vi "ATE_RVP8_Cal_Attn.vi"() -> ()   [LabVIEW 2009]
doc: "Use this template to build a producer/consumer design pattern with events to produce queue items. Use this design pattern instead of the User Interface Event Handler pattern for user interfaces when you want to execute code asynchronously in response to an event without slowing the user interface responsiveness."
uses:
  Rvp8PowerData.ctl
  <vilib>/Analysis/NI_AALBase.lvlib
  <vilib>/Analysis/NI_AALPro.lvlib
panel:
  in  "Configuration 1":bool
  out "Cal Output File":path
  out "Cal differences":cluster{i32[], dbl[]}[](graph)
  out "RVP8 calibration":cluster{i32[], dbl[]}[](graph)
  in  "DataSource":bool
  out "Cal file name":string
  in  "Cal data directory":string="/home/operator/data/rvp8_cal_attn"
  in  "Set SigGen":bool
  in  "Initialize":bool
  in  "70 dB":bool
  in  "121 dB":bool
  in  "Switches":bool
  in  "Calibrate":bool
  in  "Stop":bool
  in  "ATE TABS":enum32{"Status", "Controls"}(tab)=enum."Controls"
  out "ATE Switch Status":T1
  out "121dB\nAttenuators":bool[](array[boolean])
  out "70dB\nAttenuators":bool[](array[boolean])
  out "RVP8 Power":T2 {"time" format="%<%H:%M:%S\n%Y/%m/%d>T"}
  out "Signal Generator Status":T3={"Frequency (GHz)"=0.0, "RF Power (dBm)"=0.0, "RF Power"=TRUE} {"RF Power (dBm)" format="%.2g"}
  out "121 Verified":bool
  out "70 Verfied":bool
  in  "Start Attn dB":i32 min=0 max=121 step=1
  in  "Steps":i32=51
  in  "Steps Size dB":i32=2 min=1 max=2 step=1
  in  "RF Power (dBm)":dbl=-6.0
  in  "70 dB Attn":i32=70 min=0 max=70 step=10
  in  "121 dB Attn":i32=121 min=0 max=121 step=1
  in  "ATE Switches":T4
  out "P-State":string
  out "C-State":string
  # "RVP8 Cal - Attenuator"
  # "1 dB"
  # "2 dB"
  # "4 dB"
  # "4 dB"
  # "10 dB"
  # "20 dB"
  # "40 dB"
  # "40 dB"
  # "10 dB"
  # "20 dB"
  # "40 dB"
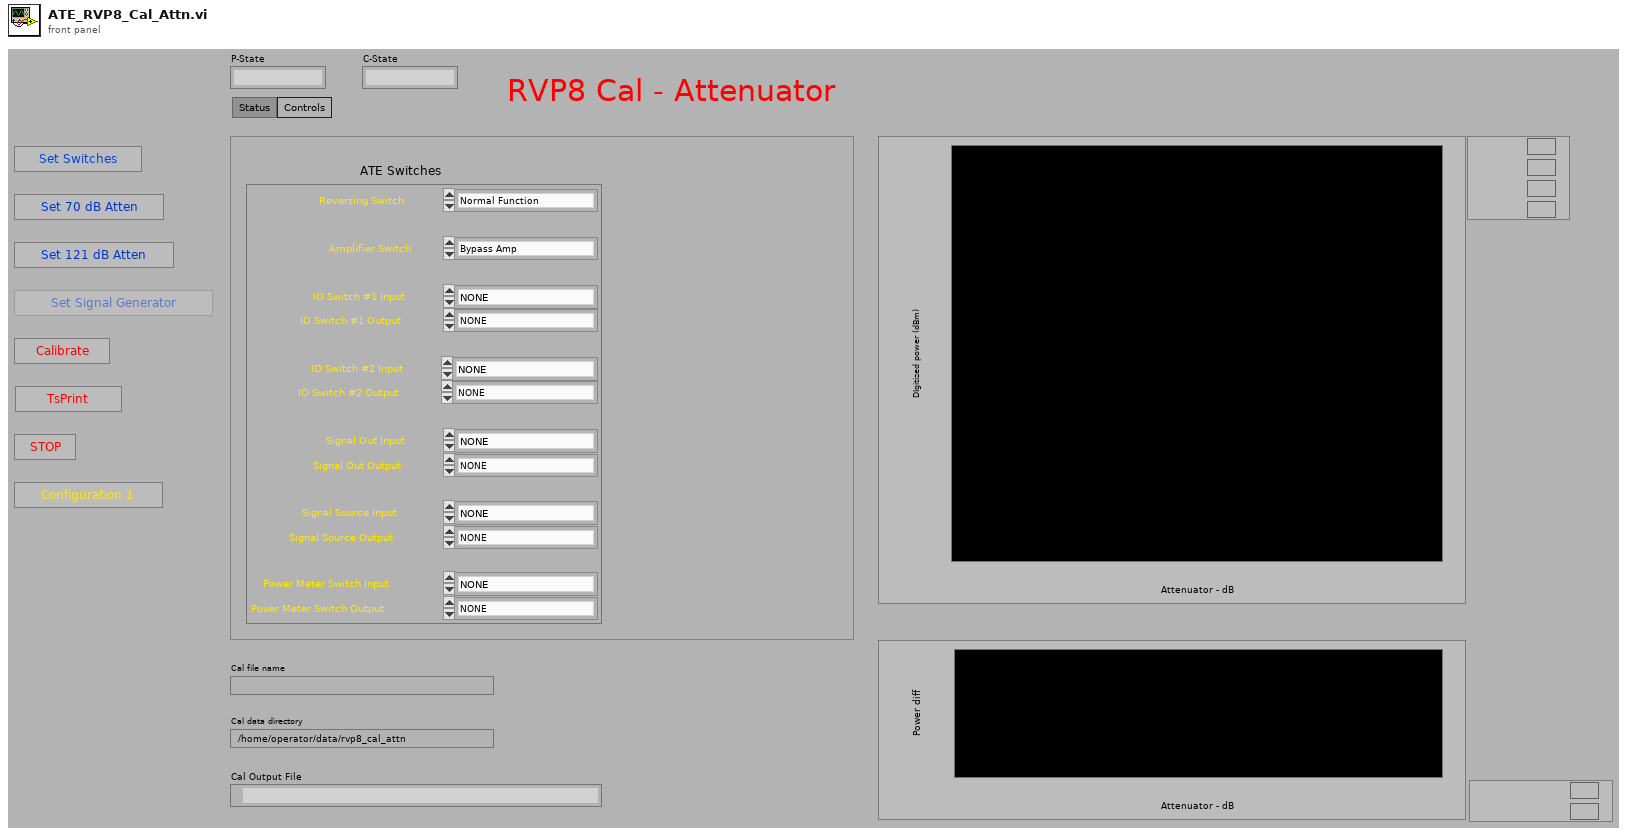
[diagram p1: front panel]
types:
  T1 = cluster{"Reversing Switch ":bool, "IO Switch #1":bool, "IO Switch #2":bool, "Signal Out":bool, "Signal Source":bool, "Power Meter":bool, "Amp By Pass":bool}
  T2 = typedef "Rvp8PowerData.ctl" = cluster{"success":bool, "time":dbl, "el":dbl, "az":dbl, "dbm0":dbl, "dbm1":dbl, "dbmHc":dbl, "dbmHx":dbl, "dbmVc":dbl, "dbmVx":dbl}
  T3 = cluster{"Frequency (GHz)":dbl, "RF Power (dBm)":dbl, "RF Power":bool}
  T4 = cluster{"Reversing Switch":enum16{"Normal Function", "Reversing Function"}, "IO Switch #1 Input":enum16{"NONE", "AHR (J2)", "Splitter", "Signal Out Switch (S3)", "Reversing Switch"}, "IO Switch #1 Output":enum16{"NONE", "AHR (J2)", "Delay Device (S4)", "Power Meter Switch (S5)", "Reversing Switch"}, "IO Switch #2 Input":enum16{"NONE", "AVR (J3)", "Splitter", "Signal Out Switch (S3)", " 2W Term (TM1)", "Reversing Switch"}, "IO Switch #2 Output":enum16{"NONE", "AVR (J3)", "Signal Out Switch (S3)", "Power Meter Switch (S5)", "Reversing Switch", "2W Term (TM1)"}, "Signal Out Input":enum16{"NONE", "Amp Bypass Switch (S6)", "IO Switch #1 (S1)", "IO Switch #2 (S2)", "2W Term (TM3)"}, "Signal Out Output":enum16{"NONE", "2 Watt Term (TM3)", "Splitter", "Power Meter Switch (S5)"}, "Signal Source Input":enum16{"NONE", "Delay Device", "Signal Generator (J7)", "Inside Noise Box NF (J5)", "2W Term (TM3)"}, "Signal Source Output":enum16{"NONE", "Amp Bypass Switch", "Test Pulse Generator", "Power Meter Switch (S5)"}, "Power Meter Switch Input":enum16{"NONE", "IO Switch #1 (S1)", "Signal Source Switch (S4)", "Signal Out Switch (S3)", "IO Switch #2 (S2)", "TXH-TXV Switch (J8)"}, "Pouer Meter Switch Output":enum16{"NONE", "Power Meter (J6)"}, "Amplifier Switch":enum16{"Bypass Amp", "Include Amp"}}
  T5 = cluster{"Frequency (GHz)":dbl, "RF Power (dBm)":dbl, "RF ON/OFF":bool}
  T6 = enum16{"open", "replace", "create", "open or create", "replace or create", "replace or create with confirmation"}
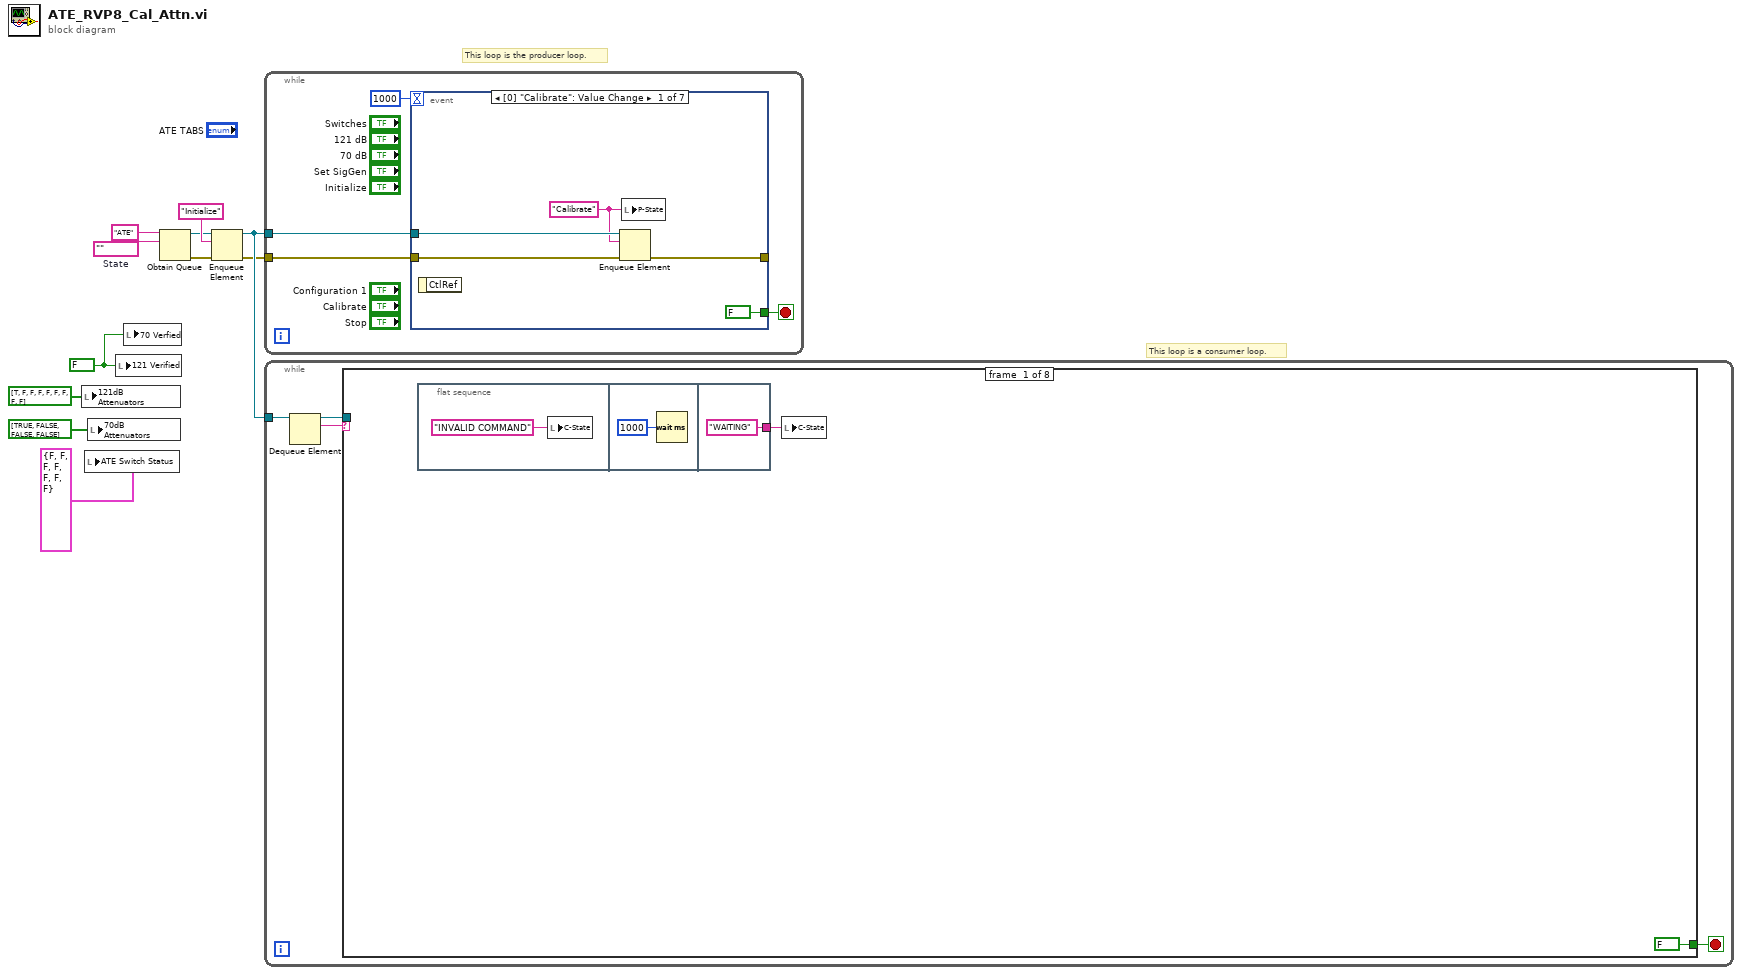
[diagram p0: block diagram]
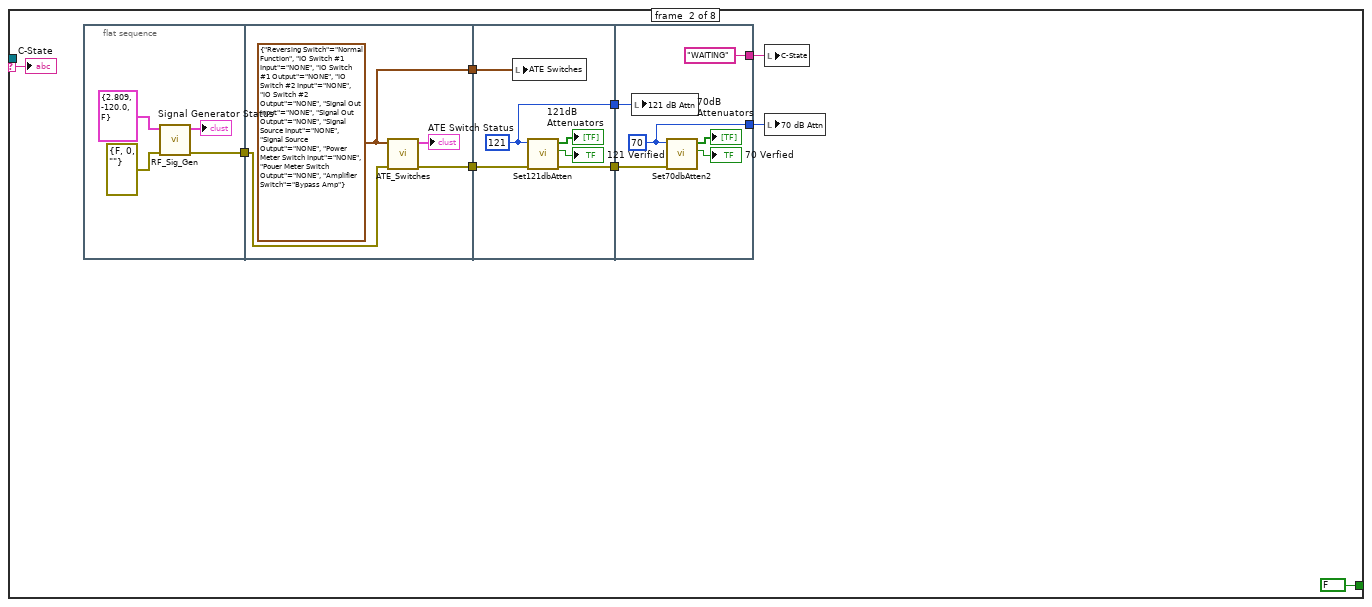
[diagram p2: hidden frame]
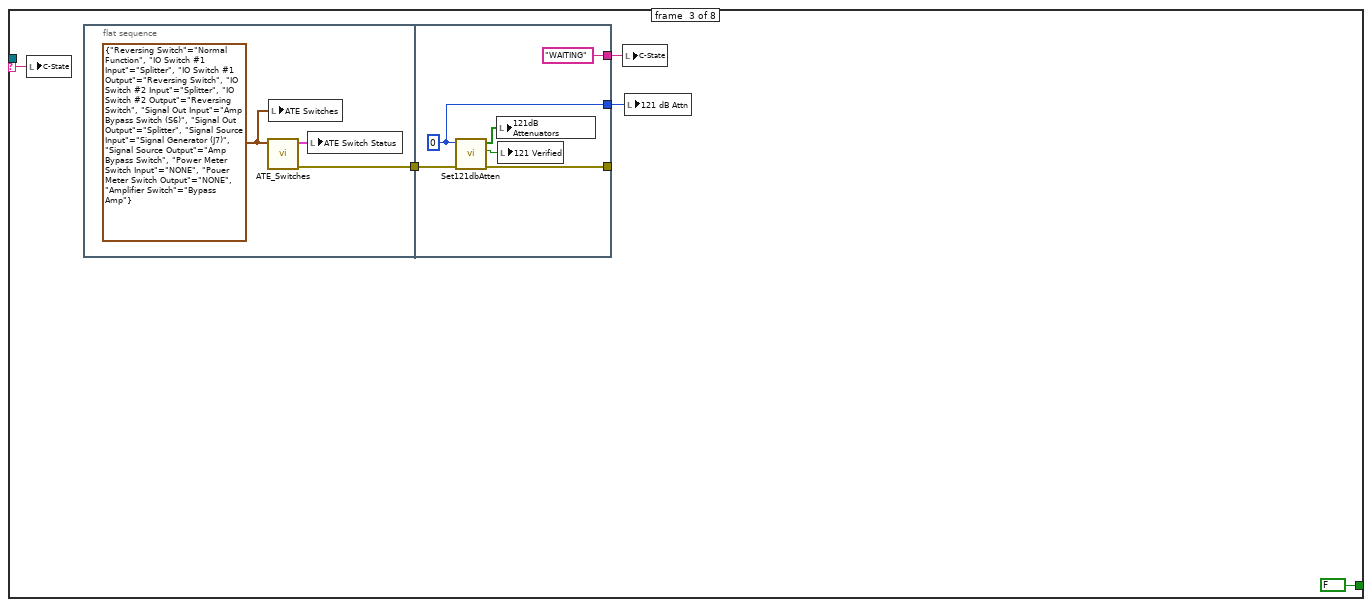
[diagram p3: hidden frame]
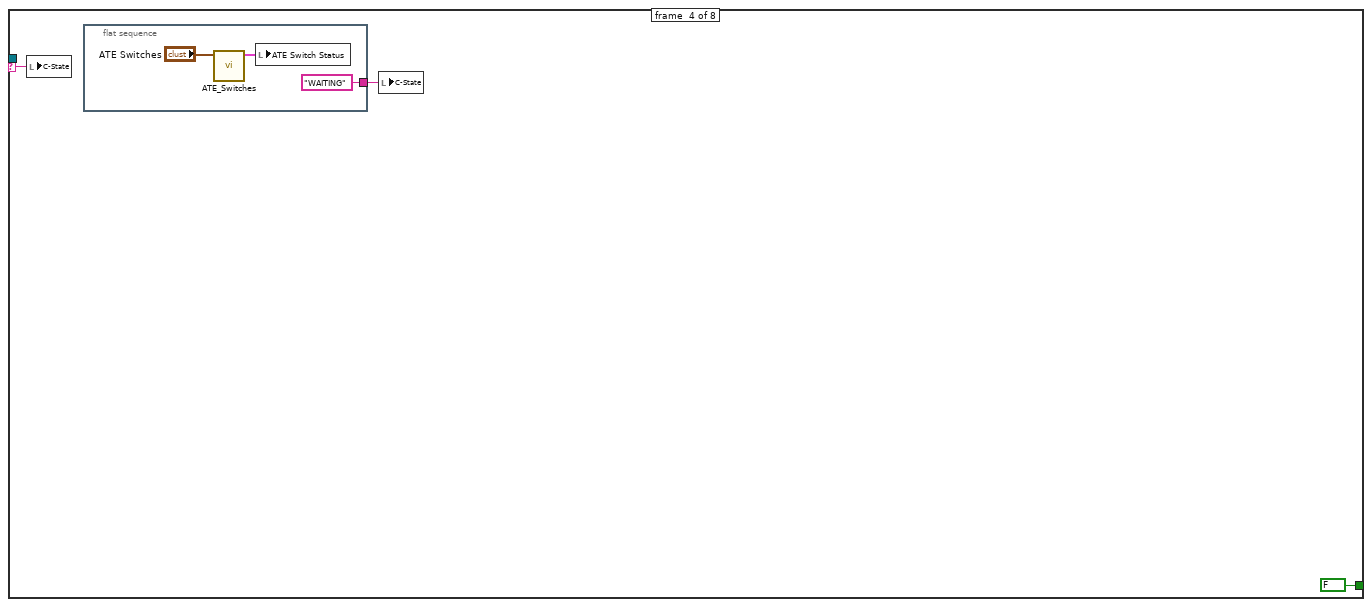
[diagram p4: hidden frame]
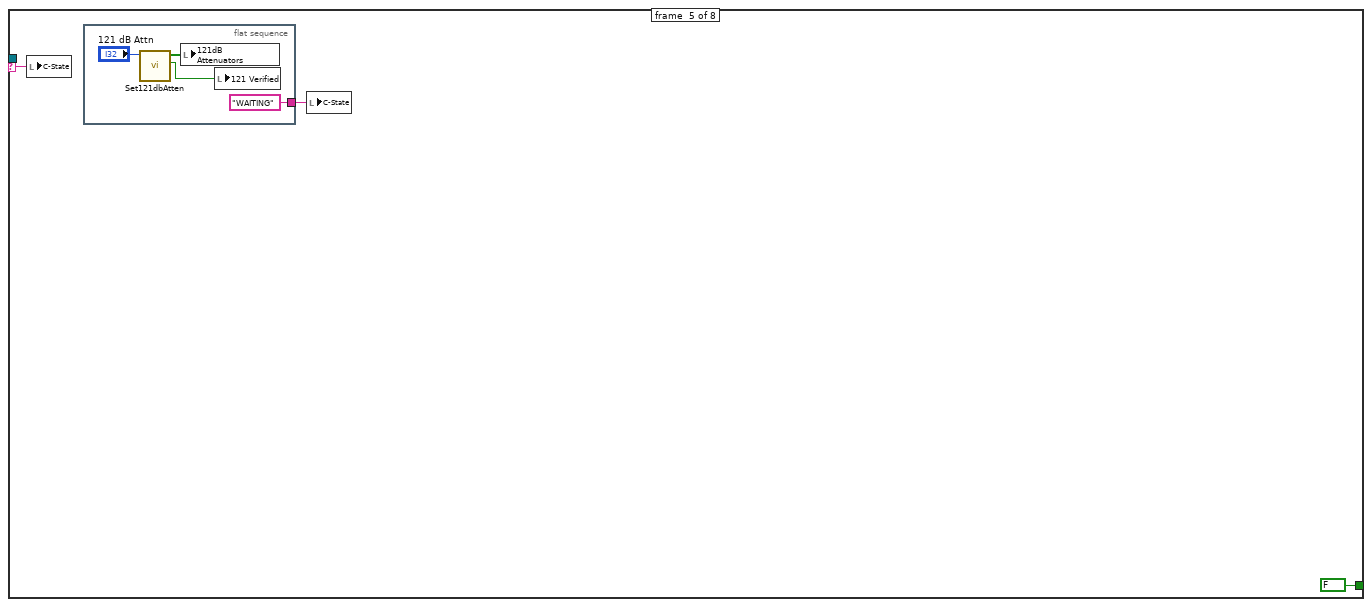
[diagram p5: hidden frame]
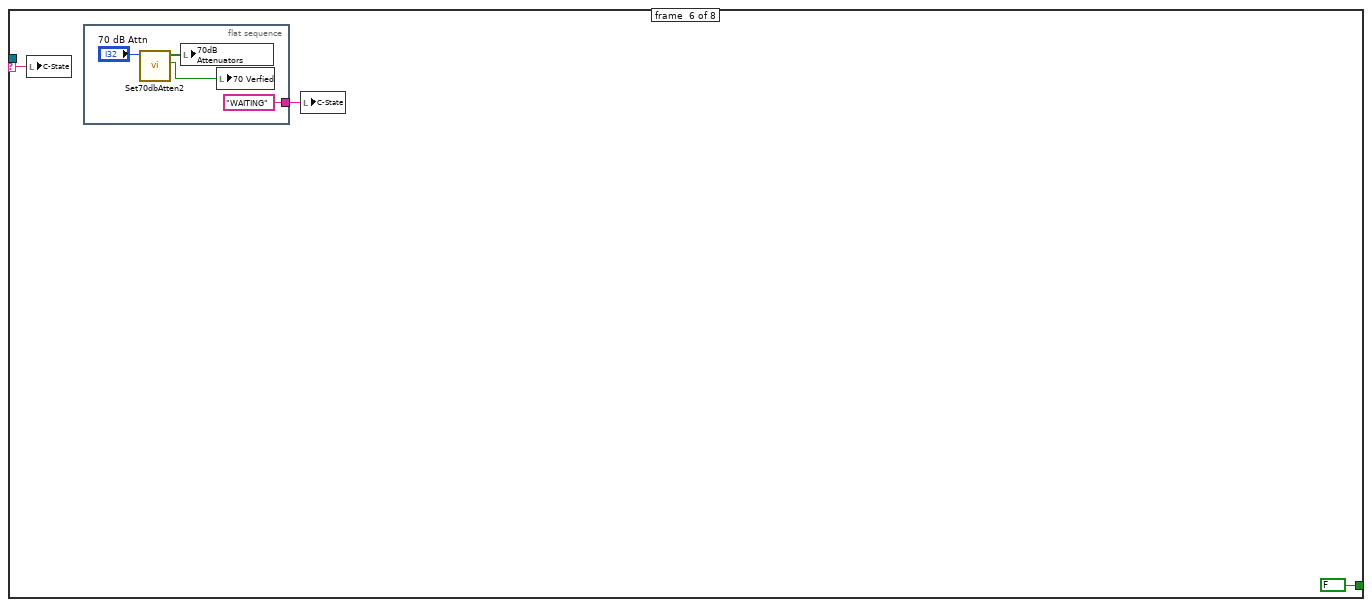
[diagram p6: hidden frame]
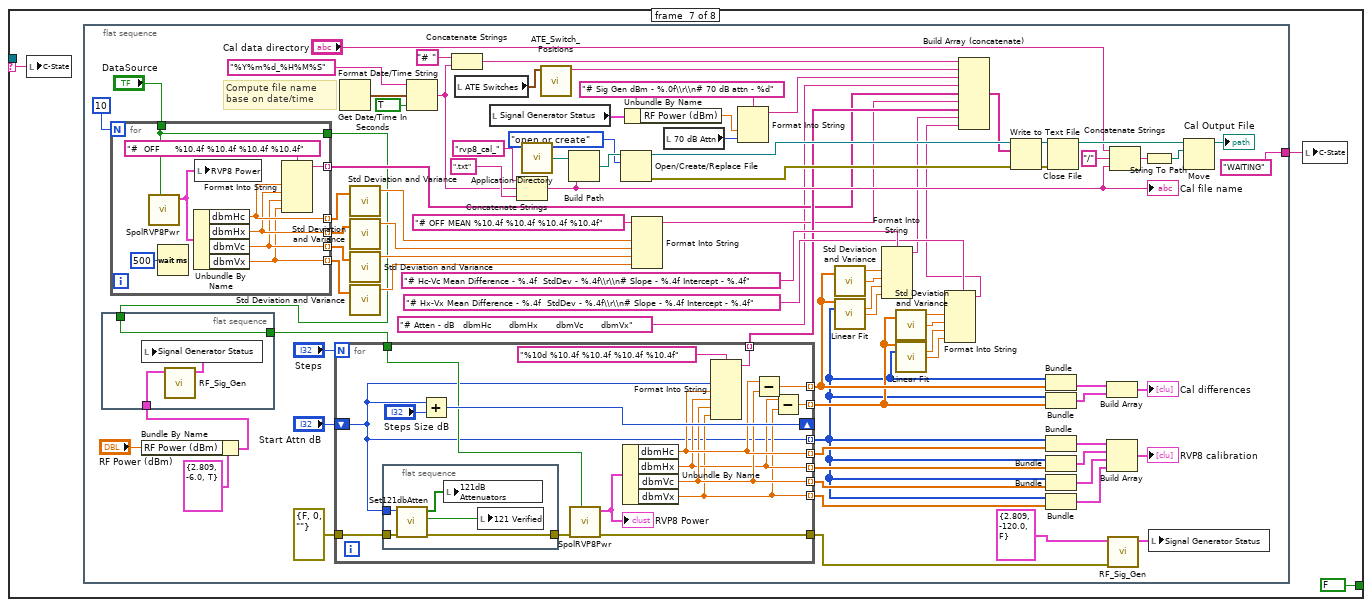
[diagram p7: hidden frame]
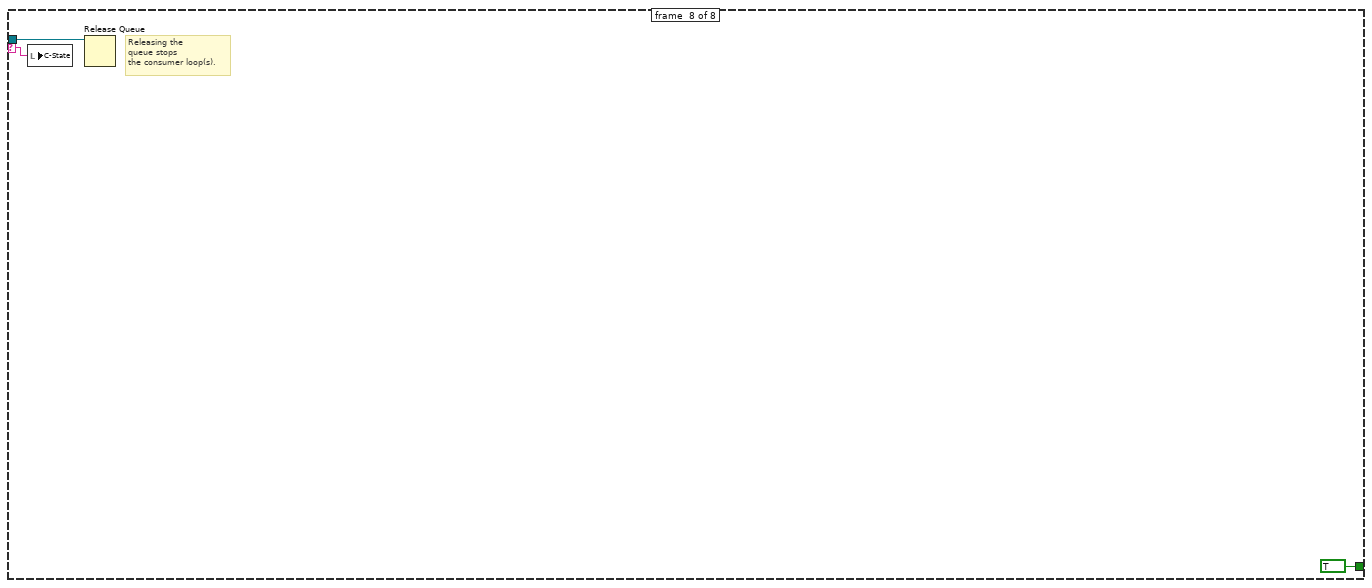
[diagram p8: hidden frame]
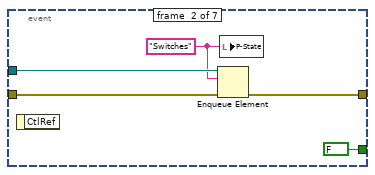
[diagram p9: hidden frame]
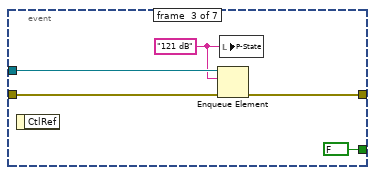
[diagram p10: hidden frame]
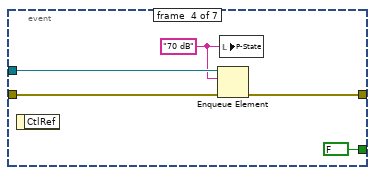
[diagram p11: hidden frame]
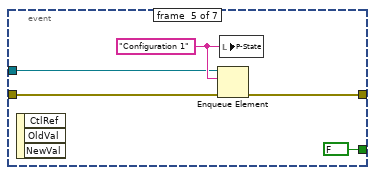
[diagram p12: hidden frame]
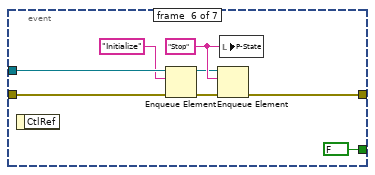
[diagram p13: hidden frame]
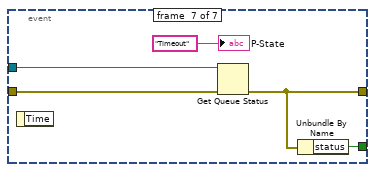
[diagram p14: hidden frame]
diagram:
  w1 = FALSE ("70 Verfied")
  w11 = ""  # State
  # "This loop is the producer loop."
  # "This loop is a consumer loop."
  n1 = local write "121dB\nAttenuators"(bool[] [TRUE, FALSE, FALSE, FALSE, FALSE, FALSE, FALSE, FALSE, FALSE] ("121dB\nAttenuators")) -> ()
  n2 = local write "ATE Switch Status"(T1 {"Reversing Switch "=FALSE, "IO Switch #1"=FALSE, "IO Switch #2"=FALSE, "Signal Out"=FALSE, "Signal Source"=FALSE, "Power Meter"=FALSE, "Amp By Pass"=FALSE} ("ATE Switch Status")) -> ()
  n3 = local write "70dB\nAttenuators"(bool[] [TRUE, FALSE, FALSE, FALSE] ("70dB\nAttenuators")) -> ()
  n4 = local write "121 Verified"(w1) -> ()
  n5 = local write "70 Verfied"(w1) -> ()
  n6 = Obtain Queue(name (unnamed)="ATE", element data type=w11) -> (queue out=w8:refnum<queue>, error out=w6:errorcluster)  [unwired: 3 in, 1 out]
  n7 = Enqueue Element(queue=w8, element="Initialize", error in (no error)=w6) -> (queue out=w7:refnum<queue>, error out=w5:errorcluster)  [unwired: 1 in, 1 out]
  n8 = while {
    tunnel: w7 -> [w15]
    tunnel: w5 -> [w14]
    stop <- w12 stop-if-true
    n9 = event shown="[0] \"Calibrate\": Value Change" {
      selector: _ -> [_ _ _ _ _ _ _]
      dyn-events: _ -> [_ _ _ _ _ _ _]
      timeout: 1000 -> [_ _ _ _ _ _ _]
      tunnel: w15 -> [w20 w25 w30 w35 w39 w43 w53]
      tunnel: w14 -> [w19 w24 w29 w34 w38 w45 w49]
      tunnel: [w18 w23 w28 w33 w37 w48 w51] -> _
      tunnel: [FALSE FALSE FALSE FALSE FALSE ("status") FALSE w52] -> w12
      event #0 {
        w16 = "Calibrate" ("element")
        n10 = event-data() -> ()  [unwired: 1 in, 1 out]
        n11 = Enqueue Element(queue=w20, element=w16, error in (no error)=w19) -> (error out=w18:errorcluster)  [unwired: 1 in, 2 out]
        n12 = local write "P-State"(w16) -> ()
      }
      event #1 {
        w21 = "Switches" ("element")
        n13 = event-data() -> ()  [unwired: 1 in, 1 out]
        n14 = Enqueue Element(queue=w25, element=w21, error in (no error)=w24) -> (error out=w23:errorcluster)  [unwired: 1 in, 2 out]
        n15 = local write "P-State"(w21) -> ()
      }
      event #2 {
        w26 = "121 dB" ("element")
        n16 = event-data() -> ()  [unwired: 1 in, 1 out]
        n17 = Enqueue Element(queue=w30, element=w26, error in (no error)=w29) -> (error out=w28:errorcluster)  [unwired: 1 in, 2 out]
        n18 = local write "P-State"(w26) -> ()
      }
      event #3 {
        w31 = "70 dB" ("element")
        n19 = event-data() -> ()  [unwired: 1 in, 1 out]
        n20 = Enqueue Element(queue=w35, element=w31, error in (no error)=w34) -> (error out=w33:errorcluster)  [unwired: 1 in, 2 out]
        n21 = local write "P-State"(w31) -> ()
      }
      event #4 {
        w40 = "Configuration 1" ("element")
        n22 = event-data() -> ()  [unwired: 1 in, 3 out]
        n23 = Enqueue Element(queue=w39, element=w40, error in (no error)=w38) -> (error out=w37:errorcluster)  [unwired: 1 in, 2 out]
        n24 = local write "P-State"(w40) -> ()
      }
      event #5 {
        w46 = "Stop" ("element")
        n25 = event-data() -> ()  [unwired: 1 in, 1 out]
        n26 = Enqueue Element(queue=w43, element="Initialize", error in (no error)=w45) -> (queue out=w42:refnum<queue>, error out=w44:errorcluster)  [unwired: 1 in, 1 out]
        n27 = Enqueue Element(queue=w42, element=w46, error in (no error)=w44) -> (error out=w48:errorcluster)  [unwired: 1 in, 2 out]
        n28 = local write "P-State"(w46) -> ()
      }
      event #6 {
        n29 = event-data() -> ()  [unwired: 1 in, 1 out]
        n30 = Get Queue Status(queue=w53, error in (no error)=w49) -> (error out=w51:errorcluster)  [unwired: 1 in, 7 out]
        n31 = Unbundle By Name(w51) -> ("status"=w52:bool)
        "P-State" <- "Timeout" ("element")
      }
    }
  }
  n32 = while {
    tunnel: w7 -> [w57]
    stop <- w54 stop-if-true
    n33 = Dequeue Element(queue=w57) -> (queue out=w55:refnum<queue>, element=w56:string)  [unwired: 2 in, 2 out]
    n34 = case shown="\"Initialize\"" w56 {
      selector: w56 -> [_ w70 w92 w108 w113 w120 w127 w247]
      tunnel: w55 -> [_ _ _ _ _ _ _ w246]
      tunnel: [FALSE FALSE FALSE FALSE FALSE FALSE FALSE TRUE] -> w54
      frame #0 {
        n35 = flat-sequence {
          tunnel: ["WAITING" ("element")] -> w58
          frame #0 {
            n36 = local write "C-State"("INVALID COMMAND" ("C-State")) -> ()
          }
          frame #1 {
            n37 = Wait (ms)(milliseconds to wait=u32 1000) -> ()  [unwired: 1 out]
          }
          frame #2 {
          }
        }
        n38 = local write "C-State"(w58) -> ()
      }
      frame #1 {
        n39 = flat-sequence {
          tunnel: [w72] -> w64
          tunnel: [w77] -> w67
          tunnel: w64 -> [w78]
          tunnel: [w76] -> w63
          tunnel: w67 -> [w84]
          tunnel: [w83] -> w68
          tunnel: [w82] -> w66
          tunnel: w63 -> [w80]
          tunnel: ["WAITING" ("element")] -> w69
          tunnel: w68 -> [w90]
          tunnel: w66 -> [w88]
          tunnel: [w87] -> w65
          frame #0 {
            n40 = call "RF_Sig_Gen.vi"("error in"=errorcluster {"status"=FALSE, "code"=0, "source"=""}, "Signal Generator Control"=T5 {"Frequency (GHz)"=2.809, "RF Power (dBm)"=-120.0, "RF ON/OFF"=FALSE}) -> ("Sig Gen Errors"=w72:errorcluster, "Signal Generator Status"=→"Signal Generator Status":T3)  [unwired: 8 in]
          }
          frame #1 {
            w76 = T4 {"Reversing Switch"=enum."Normal Function", "IO Switch #1 Input"=enum."NONE", "IO Switch #1 Output"=enum."NONE", "IO Switch #2 Input"=enum."NONE", "IO Switch #2 Output"=enum."NONE", "Signal Out Input"=enum."NONE", "Signal Out Output"=enum."NONE", "Signal Source Input"=enum."NONE", "Signal Source Output"=enum."NONE", "Power Meter Switch Input"=enum."NONE", "Pouer Meter Switch Output"=enum."NONE", "Amplifier Switch"=enum."Bypass Amp"} ("ATE Switches")
            n41 = call "ATE_Switches.vi"("error in"=w78, "ATE Switches"=w76) -> ("Switch Errors"=w77:errorcluster, "ATE Switch Status"=→"ATE Switch Status":T1)  [unwired: 8 in]
          }
          frame #2 {
            w82 = 121 ("Attenuation (dB)")
            n42 = local write "ATE Switches"(w80) -> ()
            n43 = call "Set121dbAtten.vi"("error in (no error)"=w84, "Attenuation (dB)"=w82) -> ("error out"=w83:errorcluster, "Verfied"=→"121 Verified":bool, "Active Attenuators"=→"121dB\nAttenuators":bool[])  [unwired: 7 in]
          }
          frame #3 {
            w87 = 70 ("Attenuation (dB)")
            n44 = local write "121 dB Attn"(w88) -> ()
            n45 = call "Set70dbAtten2.vi"("error in (no error)"=w90, "Attenuation (dB)"=w87) -> ("Verfied"=→"70 Verfied":bool, "Active Attenuators"=→"70dB\nAttenuators":bool[])  [unwired: 7 in, 1 out]
          }
        }
        n46 = local write "C-State"(w69) -> ()
        n47 = local write "70 dB Attn"(w65) -> ()
        "C-State" <- w70
      }
      frame #2 {
        n48 = local write "C-State"(w92) -> ()
        n49 = flat-sequence {
          tunnel: [w99] -> w95
          tunnel: w95 -> [w105]
          tunnel: [w100] -> w94
          tunnel: ["WAITING" ("element")] -> w93
          tunnel: [w103] -> _
          frame #0 {
            w97 = T4 {"Reversing Switch"=enum."Normal Function", "IO Switch #1 Input"=enum."Splitter", "IO Switch #1 Output"=enum."Reversing Switch", "IO Switch #2 Input"=enum."Splitter", "IO Switch #2 Output"=enum."Reversing Switch", "Signal Out Input"=enum."Amp Bypass Switch (S6)", "Signal Out Output"=enum."Splitter", "Signal Source Input"=enum."Signal Generator (J7)", "Signal Source Output"=enum."Amp Bypass Switch", "Power Meter Switch Input"=enum."NONE", "Pouer Meter Switch Output"=enum."NONE", "Amplifier Switch"=enum."Bypass Amp"} ("ATE Switches")
            n50 = call "ATE_Switches.vi"("ATE Switches"=w97) -> ("Switch Errors"=w99:errorcluster, "ATE Switch Status"=w98:T1)  [unwired: 9 in]
            n51 = local write "ATE Switches"(w97) -> ()
            n52 = local write "ATE Switch Status"(w98) -> ()
          }
          frame #1 {
            w100 = 0 ("Attenuation (dB)")
            n53 = call "Set121dbAtten.vi"("error in (no error)"=w105, "Attenuation (dB)"=w100) -> ("error out"=w103:errorcluster, "Verfied"=w101:bool, "Active Attenuators"=w102:bool[])  [unwired: 7 in]
            n54 = local write "121dB\nAttenuators"(w102) -> ()
            n55 = local write "121 Verified"(w101) -> ()
          }
        }
        n56 = local write "C-State"(w93) -> ()
        n57 = local write "121 dB Attn"(w94) -> ()
      }
      frame #3 {
        n58 = local write "C-State"(w108) -> ()
        n59 = flat-sequence {
          tunnel: ["WAITING" ("element")] -> w106
          frame #0 {
            n60 = call "ATE_Switches.vi"("ATE Switches"="ATE Switches") -> ("ATE Switch Status"=w110:T1)  [unwired: 9 in, 1 out]
            n61 = local write "ATE Switch Status"(w110) -> ()
          }
        }
        n62 = local write "C-State"(w106) -> ()
      }
      frame #4 {
        n63 = local write "C-State"(w113) -> ()
        n64 = flat-sequence {
          tunnel: ["WAITING" ("element")] -> w112
          frame #0 {
            n65 = call "Set121dbAtten.vi"("Attenuation (dB)"="121 dB Attn") -> ("Verfied"=w115:bool, "Active Attenuators"=w117:bool[])  [unwired: 8 in, 1 out]
            n66 = local write "121dB\nAttenuators"(w117) -> ()
            n67 = local write "121 Verified"(w115) -> ()
          }
        }
        n68 = local write "C-State"(w112) -> ()
      }
      frame #5 {
        n69 = local write "C-State"(w120) -> ()
        n70 = flat-sequence {
          tunnel: ["WAITING" ("element")] -> w119
          frame #0 {
            n71 = call "Set70dbAtten2.vi"("Attenuation (dB)"="70 dB Attn") -> ("Verfied"=w122:bool, "Active Attenuators"=w124:bool[])  [unwired: 8 in, 1 out]
            n72 = local write "70dB\nAttenuators"(w124) -> ()
            n73 = local write "70 Verfied"(w122) -> ()
          }
        }
        n74 = local write "C-State"(w119) -> ()
      }
      frame #6 {
        n75 = local write "C-State"(w127) -> ()
        n76 = flat-sequence {
          tunnel: ["WAITING" ("element")] -> w126
          frame #0 {
            # "Compute file name base on date/time"
            n77 = flat-sequence {
              tunnel: w133 -> [w214]
              tunnel: [w214] -> w132
              tunnel: w129 -> [w213]
              frame #0 {
                n78 = call "RF_Sig_Gen.vi"("Signal Generator Control"=w213) -> ("Signal Generator Status"=w215:T3)  [unwired: 9 in, 1 out]
                n79 = local write "Signal Generator Status"(w215) -> ()
              }
            }
            n80 = for {
              N: 10 -> [_]
              tunnel: [w222] -> w137 mode=indexing
              tunnel: [w221] -> w149 mode=indexing
              tunnel: [w220] -> w150 mode=indexing
              tunnel: [w219] -> w151 mode=indexing
              tunnel: [w218] -> w152 mode=indexing
              tunnel: "DataSource" -> [w217]
              tunnel: [w217] -> w133
              n81 = call "SpolRVP8Pwr.vi"("DataSource"=w217) -> ("RVP8_power"=w216:T2)  [unwired: 7 in, 3 out]
              n82 = Wait (ms)(milliseconds to wait=u32 500) -> ()  [unwired: 1 out]
              n83 = Unbundle By Name(w216) -> ("dbmHc"=w221:dbl, "dbmHx"=w220:dbl, "dbmVc"=w219:dbl, "dbmVx"=w218:dbl)
              n84 = local write "RVP8 Power"(w216) -> ()
              n85 = Format Into String(format string="#  OFF     %10.4f %10.4f %10.4f %10.4f", w221, w220, w219, w218) -> (resulting string=w222:string)  [unwired: 2 in, 1 out]
            }
            n86 = Bundle By Name(cluster=T5 {"Frequency (GHz)"=2.809, "RF Power (dBm)"=-6.0, "RF ON/OFF"=TRUE} ("Signal Generator Control"), "RF Power (dBm)"="RF Power (dBm)") -> (w129:T5)
            n87 = for {
              N: "Steps" -> [_]
              shift-right: [w232] -> _
              shift-left: "Start Attn dB" -> [w225]
              tunnel: errorcluster {"status"=FALSE, "code"=0, "source"=""} ("error out") -> [w226]
              tunnel: [w225] -> w169 mode=indexing
              tunnel: [w231] -> w204 mode=indexing
              tunnel: [w229] -> w203 mode=indexing
              tunnel: [w230] -> w202 mode=indexing
              tunnel: [w228] -> w201 mode=indexing
              tunnel: [w240] -> w139 mode=indexing
              tunnel: [w234] -> w171 mode=indexing
              tunnel: [w233] -> w170 mode=indexing
              tunnel: [w237] -> w181
              tunnel: w132 -> [w227]
              n88 = flat-sequence {
                tunnel: w226 -> [w245]
                tunnel: [w244] -> w238
                tunnel: w225 -> [w243]
                frame #0 {
                  n89 = call "Set121dbAtten.vi"("error in (no error)"=w245, "Attenuation (dB)"=w243) -> ("error out"=w244:errorcluster, "Verfied"=w241:bool, "Active Attenuators"=w242:bool[])  [unwired: 7 in]
                  n90 = local write "121dB\nAttenuators"(w242) -> ()
                  n91 = local write "121 Verified"(w241) -> ()
                }
              }
              n92 = Add(x=w225, y="Steps Size dB") -> (x+y=w232:i32)
              n93 = call "SpolRVP8Pwr.vi"("DataSource"=w227, "error in (no error)"=w238) -> ("Comm error"=w237:errorcluster, "RVP8_power"=w239:T2)  [unwired: 6 in, 2 out]
              "RVP8 Power" <- w239
              n94 = Unbundle By Name(w239) -> ("dbmHc"=w231:dbl, "dbmHx"=w229:dbl, "dbmVc"=w230:dbl, "dbmVx"=w228:dbl)
              n95 = Format Into String(format string="%10d %10.4f %10.4f %10.4f %10.4f", w225, w231, w229, w230, w228) -> (resulting string=w240:string)  [unwired: 2 in, 1 out]
              n96 = Subtract(x=w231, y=w230) -> (x-y=w234:dbl)
              n97 = Subtract(x=w229, y=w228) -> (x-y=w233:dbl)
            }
            n98 = Get Date/Time In Seconds() -> (seconds since 1Jan1904=w207:timestamp)
            n99 = call <vilib>:"Std Deviation and Variance.vi"("X"=w149) -> ("mean"=w144:dbl)  [unwired: 1 in, 2 out]
            n100 = call <vilib>:"Std Deviation and Variance.vi"("X"=w150) -> ("mean"=w143:dbl)  [unwired: 1 in, 2 out]
            n101 = call <vilib>:"Std Deviation and Variance.vi"("X"=w151) -> ("mean"=w142:dbl)  [unwired: 1 in, 2 out]
            n102 = call <vilib>:"Std Deviation and Variance.vi"("X"=w152) -> ("mean"=w145:dbl)  [unwired: 1 in, 2 out]
            n103 = Format Date/Time String(time format string (%c)="%Y%m%d_%H%M%S", seconds (now)=w207, UTC format=TRUE) -> (date/time string=w161:string)
            n104 = Concatenate Strings("# " ("string"), w161) -> (w160:string)
            n105 = local read "ATE Switches"() -> (w179:T4)
            n106 = local read "Signal Generator Status"() -> (w135:T3)
            n107 = Concatenate Strings("rvp8_cal_", w161, ".txt") -> (w157:string)
            "Cal file name" <- w157
            n108 = call <vilib>:"Application Directory.vi"() -> ("Application Directory"=w206:path)
            n109 = call "ATE_Switch_Positions.vi"("ATE Switches"=w179) -> ("ATE Switch/Position"=w159:string)  [unwired: 10 in]
            n110 = Build Path(base path=w206, name or relative path=w157) -> (appended path=w192:path)
            n111 = Open/Create/Replace File(file path (use dialog)=w192, operation (0:open)=T6."open or create") -> (refnum out=w191:refnum<file>, error out=w190:errorcluster)  [unwired: 4 in, 1 out]
            n112 = Unbundle By Name(w135) -> ("RF Power (dBm)"=w134:dbl)
            n113 = Format Into String(format string="# OFF MEAN %10.4f %10.4f %10.4f %10.4f", w144, w143, w142, w145) -> (resulting string=w138:string)  [unwired: 2 in, 1 out]
            n114 = local read "70 dB Attn"() -> (w176:i32)
            n115 = Format Into String(format string="# Sig Gen dBm - %.0f\\r\\n# 70 dB attn - %d", w134, w176) -> (resulting string=w158:string)  [unwired: 2 in, 1 out]
            n116 = call <vilib>:"Std Deviation and Variance.vi"("X"=w171) -> ("mean"=w175:dbl, "standard deviation"=w172:dbl)  [unwired: 1 in, 1 out]
            n117 = call <vilib>:"Linear Fit.vi"("Y"=w171, "X"=w169) -> ("slope"=w174:dbl, "intercept"=w173:dbl)  [unwired: 9 in, 3 out]
            n118 = Format Into String(format string="# Hc-Vc Mean Difference - %.4f  StdDev - %.4f\\r\\n# Slope - %.4f Intercept - %.4f", w175, w172, w174, w173) -> (resulting string=w140:string)  [unwired: 2 in, 1 out]
            n119 = call <vilib>:"Std Deviation and Variance.vi"("X"=w170) -> ("mean"=w168:dbl, "standard deviation"=w167:dbl)  [unwired: 1 in, 1 out]
            n120 = call <vilib>:"Linear Fit.vi"("Y"=w170, "X"=w169) -> ("slope"=w166:dbl, "intercept"=w165:dbl)  [unwired: 9 in, 3 out]
            n121 = Format Into String(format string="# Hx-Vx Mean Difference - %.4f  StdDev - %.4f\\r\\n# Slope - %.4f Intercept - %.4f", w168, w167, w166, w165) -> (resulting string=w141:string)  [unwired: 2 in, 1 out]
            n122 = Build Array (concatenate)(w160, w159, w158, "# Atten - dB   dbmHc      dbmHx      dbmVc      dbmVx", w137, w138, w139, w140, w141) -> (w178:string[])
            n123 = Write to Text File(file (use dialog)=w191, text=w178, error in=w190) -> (refnum out=w189:refnum<file>, error out=w188:errorcluster)  [unwired: 1 in, 1 out]
            n124 = Bundle(w169, w171) -> (w200:cluster{i32[], dbl[]})  [unwired: 1 in]
            n125 = Bundle(w169, w170) -> (w199:cluster{i32[], dbl[]})  [unwired: 1 in]
            n126 = Bundle(w169, w204) -> (w198:cluster{i32[], dbl[]})  [unwired: 1 in]
            n127 = Bundle(w169, w203) -> (w197:cluster{i32[], dbl[]})  [unwired: 1 in]
            n128 = Bundle(w169, w202) -> (w195:cluster{i32[], dbl[]})  [unwired: 1 in]
            n129 = Bundle(w169, w201) -> (w196:cluster{i32[], dbl[]})  [unwired: 1 in]
            n130 = Close File(refnum=w189, error in=w188) -> (path=w185:path)  [unwired: 1 out]
            n131 = Build Array(w200, w199) -> (→"Cal differences":cluster{i32[], dbl[]}[])
            n132 = Build Array(w198, w197, w195, w196) -> (→"RVP8 calibration":cluster{i32[], dbl[]}[])
            n133 = call "RF_Sig_Gen.vi"("error in"=w181, "Signal Generator Control"=T5 {"Frequency (GHz)"=2.809, "RF Power (dBm)"=-120.0, "RF ON/OFF"=FALSE}) -> ("Signal Generator Status"=w182:T3)  [unwired: 8 in, 1 out]
            n134 = Concatenate Strings("Cal data directory", "/" ("string"), w157) -> (w186:string)
            n135 = String To Path(string=w186) -> (path=w184:path)
            n136 = local write "Signal Generator Status"(w182) -> ()
            n137 = Move(source path=w185, 10:w184) -> (3:→"Cal Output File":path)  [unwired: 3 in, 2 out]
          }
        }
        n138 = local write "C-State"(w126) -> ()
      }
      frame #7 {
        # "Releasing the\nqueue stops\nthe consumer loop(s)."
        n139 = local write "C-State"(w247) -> ()
        n140 = Release Queue(queue=w246) -> ()  [unwired: 2 in, 3 out]
      }
    }
  }
